vi "Dendrites detection plugin.vi"(7 "ROI":T2, 9 "Function":T1, 11 "16 bit image in":T3=refnum) -> (0 "Nb Circles last iteration":i32, 1 "Skipped":bool, 2 "Circles Data":T4(array[cluster]), 3 "Nb Circles":i32)   [LabVIEW 2017]
uses:
  <vilib>/vision/Image Controls.llb/IMAQ Image.ctl
  Typedefs/Duplicate POI function enum.ctl
  Globals/gl_ROI Entry UI globals.vi
  <vilib>/vision/NI_Vision_Development_Module.lvlib
panel:
  out "Image":T3(plugin-control)
  out "Masked":T3(plugin-control)
  out "Exposed somas":T3(plugin-control)
  out "somas subtracted":T3(plugin-control)
  out "AutoM":T3(plugin-control)
  out "Upper class only":T3(plugin-control)
  out "Classes":T3(plugin-control)
  in  "Min Radius":sgl=2.0
  in  "Max Radius":sgl=10.0
  out "Circles":T3(plugin-control)
  in  "Number of Classes":i32=2 min=2 max=30 step=1
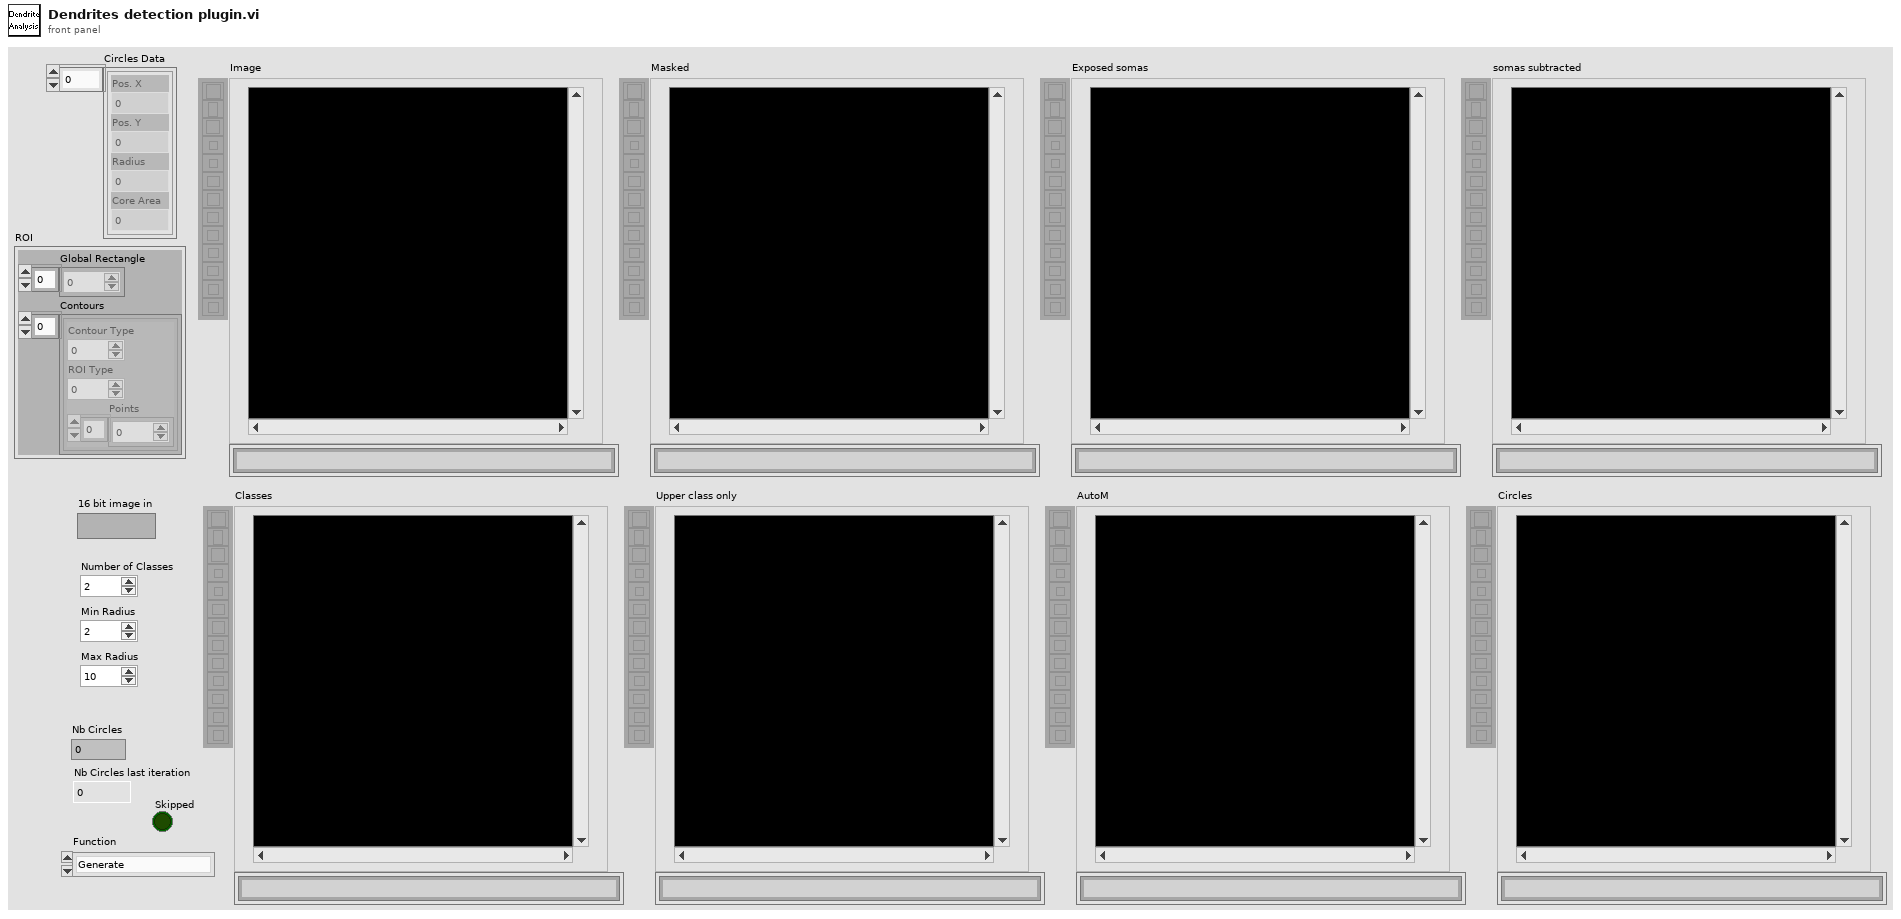
[diagram p1: front panel]
types:
  T1 = typedef "Duplicate POI function enum.ctl" = enum16{"Generate", "Adjust number of POI", "Clear register"}
  T2 = cluster{"Global Rectangle":i32[], "Contours":cluster{"Contour Type":u32, "ROI Type":u32, "Points":i32[]}[]}
  T3 = typedef "IMAQ Image.ctl" = refnum<image>
  T4 = cluster{"Pos. X":i32, "Pos. Y":i32, "Radius":i32, "Core Area":i32}[]
  T5 = typedef "ROI entry screen ctrl refs cluster.ctl" = cluster{"Done button":refnum<vi>, "Imaging button":refnum<vi>, "Acquisition button":refnum<vi>, "POI dwell time (us)":refnum<vi>, "Scan dwell time per pixel (us)":refnum<vi>, "# of planes":refnum<vi>, "Zoom Ctrl":refnum<vi>, "Equal size":refnum<vi>, "Channel":refnum<vi>, "Image Display":refnum<vi>, "Z-Plane Selector":refnum<vi>, "Number of lines left":refnum<vi>, "Z-stack folder path":refnum<vi>, "POI Density":refnum<vi>, "Arb Plane Entry":refnum<vi>, "Whole plane":refnum<vi>, "Clear Last":refnum<vi>, "Clear All":refnum<vi>, "Trial Length (sec)":refnum<vi>, "Palette Type":refnum<vi>, "Intensity slider":refnum<vi>, "# POI":refnum<vi>, "Max Z Proj":refnum<vi>, "Zplane ind":refnum<vi>, "Wavelength (nm)":refnum<vi>, "Number of Trials":refnum<vi>, "Funct stim.trig.enable":refnum<vi>, "Funct stim.trig.delay (s)":refnum<vi>, "Line Mode":refnum<vi>, "Step size (µm)":refnum<vi>, "ROI move mode":refnum<vi>, "Cool-down time (s)":refnum<vi>, "Enable cool-down time":refnum<vi>, "Motor Z ind. (um)":refnum<vi>, "AOL Z ind. (um)":refnum<vi>, "Load Reference Image":refnum<vi>}
  T6 = enum32{"AutoM", "Close", "Dilate", "Erode", "Gradient", "Gradient out", "Gradient in", "Hit miss", "Open", "PClose", "POpen", "Thick", "Thin"}
  T7 = typedef "Image Type" = u32
  T8 = cluster{"Lower value":sgl, "Upper value":sgl, "Replace Value":sgl, "Keep/Replace Value (Replace)":bool}[]
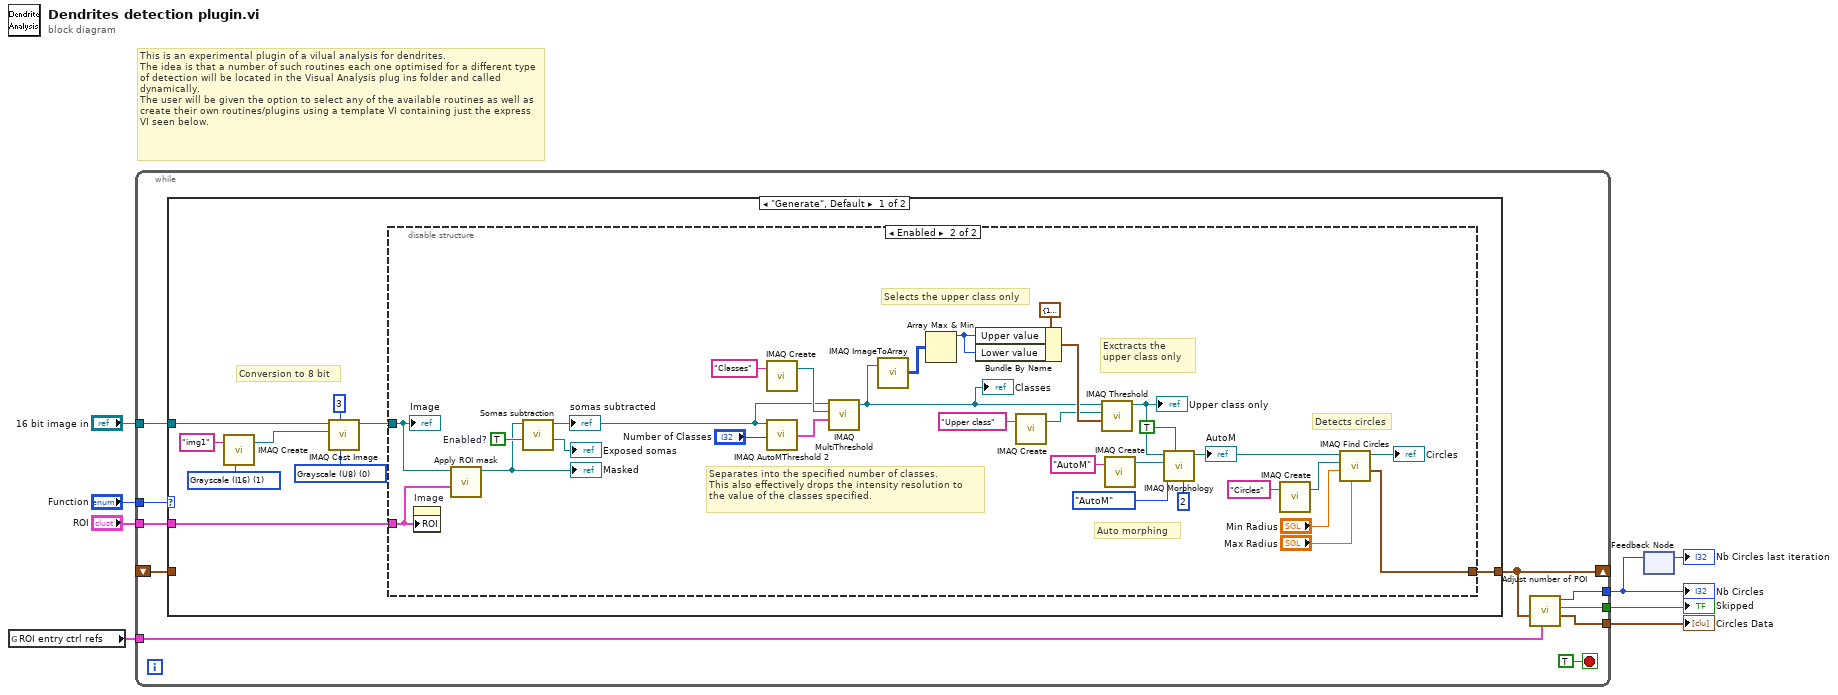
[diagram p0: block diagram]
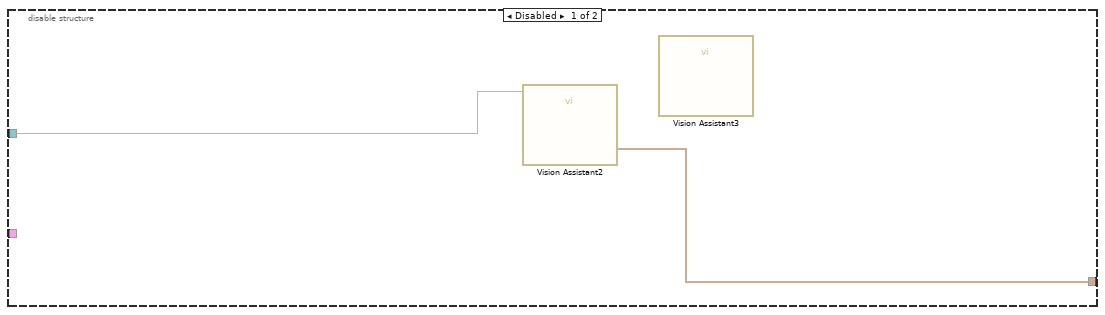
[diagram p2: hidden frame]
diagram:
  # "This is an experimental plugin of a vilual analysis for dendrites.\nThe idea is that a number of such routines each one optimised for a different type of detection will be located in the Visual Analysis plug ins folder and called dynamically.\nThe user will be given the option to select any of the available routines as well as create their own routines/plugins using a template VI containing just the express VI seen below."
  n1 = global read "gl_ROI Entry UI globals.vi" "ROI entry ctrl refs"() -> (w1:T5)
  n2 = while {
    tunnel: "16 bit image in" -> [w18]
    tunnel: "ROI" -> [w17]
    tunnel: "Function" -> [w16]
    shift-right: [w12] -> _
    shift-left: _ -> [w15]
    tunnel: [w13] -> w5
    tunnel: [w11] -> w3
    tunnel: [w10] -> w4
    tunnel: w1 -> [w9]
    stop <- TRUE stop-if-true
    n3 = case shown="\"Generate\", Default" w16 {
      tunnel: [w27 w60] -> w12
      tunnel: w18 -> [w21 _]
      tunnel: w17 -> [w19 _]
      tunnel: w15 -> [_ w60]
      frame "Generate", Default {
        w22 = T7 0 items=["Grayscale (U8)", "Grayscale (I16)", "Grayscale (SGL)", "Complex (CSG)", "RGB (U32)", "HSL (U32)", "RGB (U64)", "Grayscale (U16)"] ("Image Type")
        w26 = T7 1 items=["Grayscale (U8)", "Grayscale (I16)", "Grayscale (SGL)", "Complex (CSG)", "RGB (U32)", "HSL (U32)", "RGB (U64)", "Grayscale (U16)"] ("Image Type")
        # "Conversion to 8 bit"
        n4 = call "IMAQ Create"("Image Name"="img1", "Image Type"=w26) -> ("New Image"=w24:T3)  [unwired: 3 in, 1 out]
        n5 = call "IMAQ Cast Image"("Image Type"=w22, "# Shifts"=3, "Image Dst"=w24, "Image Src"=w21) -> ("Image Dst Out"=w20:T3)  [unwired: 6 in, 1 out]
        n6 = disable-structure "Diagram Disable Structure" shown="Enabled" {
          disable-tunnel: w20 -> [w29 w32]
          disable-tunnel: [w28 w30] -> w27
          disable-tunnel: w19 -> [_ w31]
          frame Disabled {
            n7 = call "Vision Assistant2"("Image In"=w29) -> ("Circles Data (Circle Detection 1)"=w28:T4)  [unwired: 23 in, 3 out]
            n8 = call "Vision Assistant3"() -> ()  [unwired: 26 in, 2 out]
          }
          frame Enabled {
            w36 = TRUE  # Enabled?
            # "Auto morphing"
            # "Selects the upper class only"
            # "Detects circles"
            # "Exctracts the upper class only"
            # "Separates into the specified number of classes.\nThis also effectively drops the intensity resolution to\nthe value of the classes specified."
            n9 = property on="Image" class="ImageControl"("ROI"=w31) -> ()  [unwired: 2 in, 2 out]
            n10 = call "Apply ROI mask.vi"("ROI"=w31, "Refnum in"=w32) -> ("Masked"=w33:T3)  [unwired: 9 in]
            "Masked" <- w33
            n11 = call "Somas subtraction.vi"("Enabled? (T)"=w36, "Input image (binary)"=w33) -> ("Exposed somas"=→"Exposed somas":T3, "somas subtracted"=w34:T3)  [unwired: 8 in]
            "somas subtracted" <- w34
            n12 = call "IMAQ Create"("Image Name"="Classes") -> ("New Image"=w56:T3)  [unwired: 4 in, 1 out]
            n13 = call "IMAQ AutoMThreshold 2"("Number of Classes"="Number of Classes", "Image"=w34) -> ("Threshold Data out"=w59:T8)  [unwired: 2 in, 2 out]
            n14 = call "IMAQ MultiThreshold"("Threshold Data"=w59, "Image Dst"=w56, "Image Src"=w34) -> ("Image Dst Out"=w38:T3)  [unwired: 2 in, 1 out]
            "Classes" <- w38
            n15 = call "IMAQ ImageToArray"("Image"=w38) -> ("Image Pixels (U8)"=w55:u8[][])  [unwired: 3 in, 4 out]
            n16 = Array Max & Min(array=w55) -> (max value=w52:u8)  [unwired: 3 out]
            n17 = Bundle By Name(cluster=cluster{"Lower value":sgl, "Upper value":sgl} {"Lower value"=128.0, "Upper value"=255.0} ("Range"), "Upper value"=w52, "Lower value"=w52) -> (w53:cluster{"Lower value":sgl, "Upper value":sgl})
            n18 = call "IMAQ Create"("Image Name"="Upper class") -> ("New Image"=w45:T3)  [unwired: 4 in, 1 out]
            n19 = call "IMAQ Threshold"("Range"=w53, "Image Dst"=w45, "Image Src"=w38) -> ("Image Dst Out"=w39:T3)  [unwired: 7 in, 1 out]
            "Upper class only" <- w39
            n20 = call "IMAQ Create"("Image Name"="AutoM") -> ("New Image"=w43:T3)  [unwired: 4 in, 1 out]
            n21 = call "IMAQ Morphology"("Number of iterations (1)"=2, "Square/Hexa (Square)"=TRUE, "Operation"=T6."AutoM", "Image Dst"=w43, "Image Src"=w39) -> ("Image Dst Out"=w35:T3)  [unwired: 5 in, 1 out]
            "AutoM" <- w35
            n22 = call "IMAQ Create"("Image Name"="Circles") -> ("New Image"=w49:T3)  [unwired: 4 in, 1 out]
            n23 = call "IMAQ Find Circles"("Max Radius"="Max Radius", "Min Radius"="Min Radius", "Image Dst"=w49, "Image Src"=w35) -> ("Circles Data"=w30:T4, "Image Dst Out"=→"Circles":T3)  [unwired: 4 in, 2 out]
            "Image" <- w32
          }
        }
      }
      frame "Adjust number of POI" {
      }
    }
    n24 = call "Adjust number of POI.vi"("Ctrl refs"=w9, "Circles Data in"=w12) -> ("Circles Data out"=w13:T4, "Skipped"=w10:bool, "Nb Circles out"=w11:i32)  [unwired: 7 in]
  }
  "Circles Data" <- w5
  "Nb Circles" <- w3
  "Skipped" <- w4
  n25 = feedback-in #1(w3) -> ()
  n26 = feedback #1() -> (→"Nb Circles last iteration":i32)  [unwired: 1 in]
